vi "test_blank.vi"(11 "number":i32) -> ()   [LabVIEW 2020]
panel:
  out "running":i32
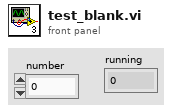
[diagram p1: front panel]
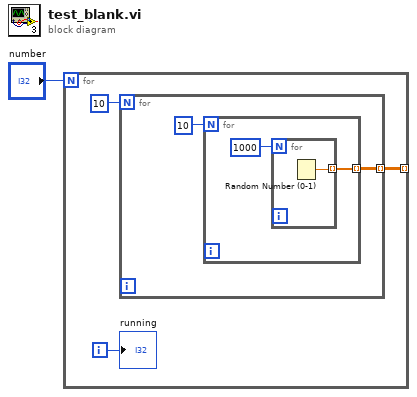
[diagram p0: block diagram]
diagram:
  n1 = for {
    N: "number" -> [_]
    tunnel: [w4] -> _ mode=indexing
    i -> [w2]
    n2 = for {
      N: 10 -> [_]
      tunnel: [w6] -> w4 mode=indexing
      n3 = for {
        N: 10 -> [_]
        tunnel: [w8] -> w6 mode=indexing
        n4 = for {
          N: 1000 -> [_]
          tunnel: [w9] -> w8 mode=indexing
          n5 = Random Number (0-1)() -> (number: 0 to 1=w9:dbl)
        }
      }
    }
    "running" <- w2
  }
